vi "Calculate Stuff.vi"(0 "RTD in":dbl[](array[numeric]), 1 "Compressor Displacement Volume":dbl, 3 "Power (Need Input Module)":dbl format="%#_13g", 5 "TC in":dbl[](array[numeric]), 7 "Units":string(combo), 9 "P in":dbl[](array[numeric]), 11 "mdot in":dbl[](array[numeric]), 12 "Compressor Rotational Speed (need input module)":dbl, 14 "fluid name":u16(ring)=17 items=["AIR.MIX", "AMARILLO.MIX", "EKOFISK.MIX", "GLFCOAST.MIX", "HIGHCO2.MIX", "HIGHN2.MIX", "NGSAMPLE.MIX", "R401A.MIX", "R401B.MIX", "R401C.MIX", "R402A.MIX", "R402B.MIX", "R403A.MIX", "R403B.MIX", "R405A.MIX", "R406A.MIX", "R407A.MIX", "R407B.MIX", "R407C.MIX", "R407D.MIX", "R407E.MIX", "R408A.MIX", "R409A.MIX", "R409B.MIX", "R410A.PPF", "R410B.MIX", "R411A.MIX", "R411B.MIX", "R412A.MIX", "R413A.MIX", "R414B.MIX", "R415A.MIX", "R415B.MIX", "R416A.MIX", "R417A.MIX", "R417B.MIX", "R417C.MIX", "R418A.MIX", "R419A.MIX", "R419B.MIX", "R420A.MIX", "R421A.MIX", "R421B.MIX", "R422A.MIX", "R422B.MIX", "R422C.MIX", "R422D.MIX", "R422E.MIX", "R423A.MIX", "R424A.MIX", "R425A.MIX", "R426A.MIX", "R427A.MIX", "R428A.MIX", "R429A.MIX", "R430A.MIX", "R431A.MIX", "R432A.MIX", "R433A.MIX", "R433B.MIX", "R433C.MIX", "R434A.MIX", "R435A.MIX", "R436A.MIX", "R436B.MIX", "R437A.MIX", "R438A.MIX", "R439A.MIX", "R440A.MIX", "R441A.MIX", "R442A.MIX", "R443A.MIX", "R444A.MIX", "R444B.MIX", "R445A.MIX", "R446A.MIX", "R447A.MIX", "R448A.MIX", "R449A.MIX", "R449B.MIX", "R450A.MIX", "R451A.MIX", "R451B.MIX", "R452A.MIX", "R452B.MIX", "R452C.MIX", "R453A.MIX", "R454A.MIX", "R454B.MIX", "R454C.MIX", "R455A.MIX", "R456A.MIX", "R457A.MIX", "R459A.MIX", "R459B.MIX", "R460A.MIX", "R460B.MIX", "R500.MIX", "R501.MIX", "R502.MIX", "R503.MIX", "R504.MIX", "R507A.MIX", "R508A.MIX", "R508B.MIX", "R509A.MIX", "R510A.MIX", "R511A.MIX", "R512A.MIX", "R513A.MIX", "R513B.MIX", "R515A.MIX", "ammonia.fld", "butane.fld", "ethane.fld", "propane.fld", "R11.fld", "R113.fld", "R114.fld", "R115.fld", "R116.fld", "R12.fld", "R123.fld", "R124.fld", "R125.fld", "R13.fld", "R134a.fld", "R14.fld", "R141b.fld", "R142b.fld", "R143a.fld", "R152a.fld", "R161.fld", "R21.fld", "R218.fld", "R22.fld", "R227ea.fld", "R23.fld", "R236ea.fld", "R236fa.fld", "R245ca.fld", "R245fa.fld", "R32.fld", "R41.fld", "R1216.fld", "RC318.fld", "water.fld", "1butene.fld", "acetone.fld", "argon.fld", "benzene.fld", "c1cc6.fld", "c2butene.fld", "c3cc6.fld", "c4f10.fld", "c5f12.fld", "c11.fld", "c12.fld", "cf3i.fld", "CO.fld", "CO2.fld", "COS.fld", "cyclohex.fld", "cyclopen.fld", "cyclopro.fld", "D2.fld", "D2O.fld", "D4.fld", "D5.fld", "D6.fld", "decane.fld", "dee.fld", "dmc.fld", "dme.fld", "ebenzene.fld", "ethanol.fld", "ethylene.fld", "flourine.fld", "H2S.fld", "HCl.fld", "helium.fld", "heptane.fld", "hexane.fld", "hydrogen.fld", "ibutene.fld", "ihexane.fld", "ioctane.fld", "ipentane.fld", "isobutan.fld", "krypton.fld", "MD2M.fld", "MD3M.fld", "MD4M.fld", "MDM.fld", "methane.fld", "methanol.fld", "mlinolea.fld", "mlinolen.fld", "MM.fld", "moleate.fld", "mpalmita.fld", "mstearat.fld", "mxylene.fld", "N2O.fld", "neon.fld", "neopentn.fld", "NF3.fld", "nitrogen.fld", "nonane.fld", "novec649.fld", "octane.fld", "orthohyd.fld", "oxygen.fld", "parahyd.fld", "pentane.fld", "propylen.fld", "propyne.fld", "pxylene.fld", "R365MFC.fld", "R1233zd.fld", "R1234yf.fld", "R1234ze.fld", "RE143a.fld", "RE245cb2.fld", "RE245fa2.fld", "RE347mcc.fld", "sf6.fld", "SO2.fld", "T2butene.fld", "xenon.fld"]) -> (4 "Calculated Values":dbl[](array[numeric]))   [LabVIEW 2017]
panel:
  out "Capacity":dbl
  out "DT subcool":dbl
  out "DT superheat":dbl
  out "Isentropic Efficiency":dbl
  out "Volumetric Efficiency":dbl
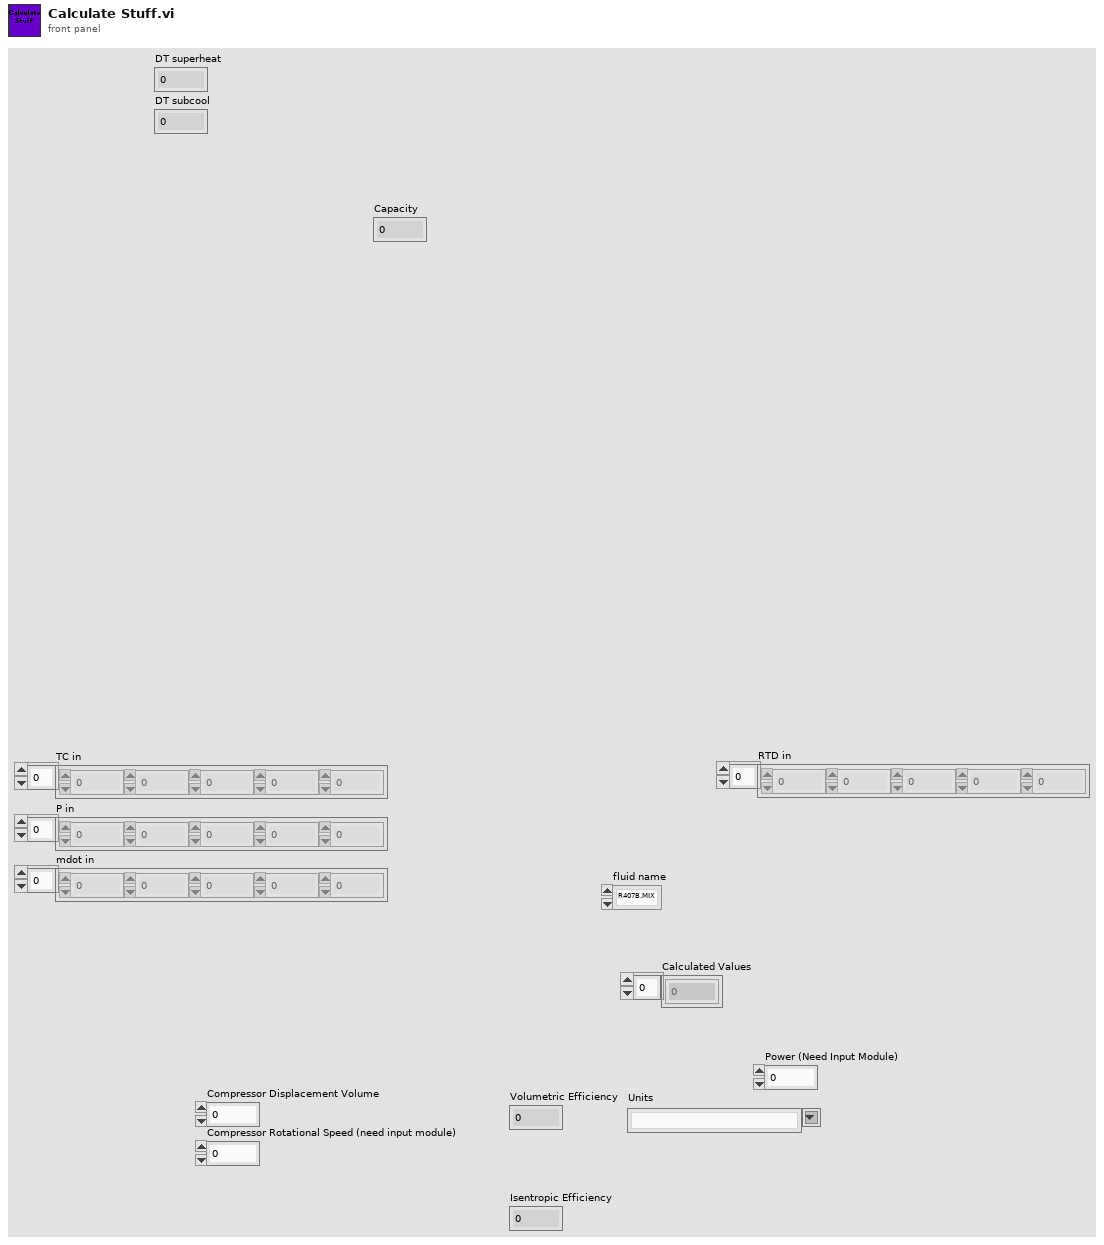
[diagram p1: front panel]
types:
  T1 = enum16{"0", "PS", "HS", "T", "P", "TP", "TH", "TS", "PH", "PQ", "TQ"}
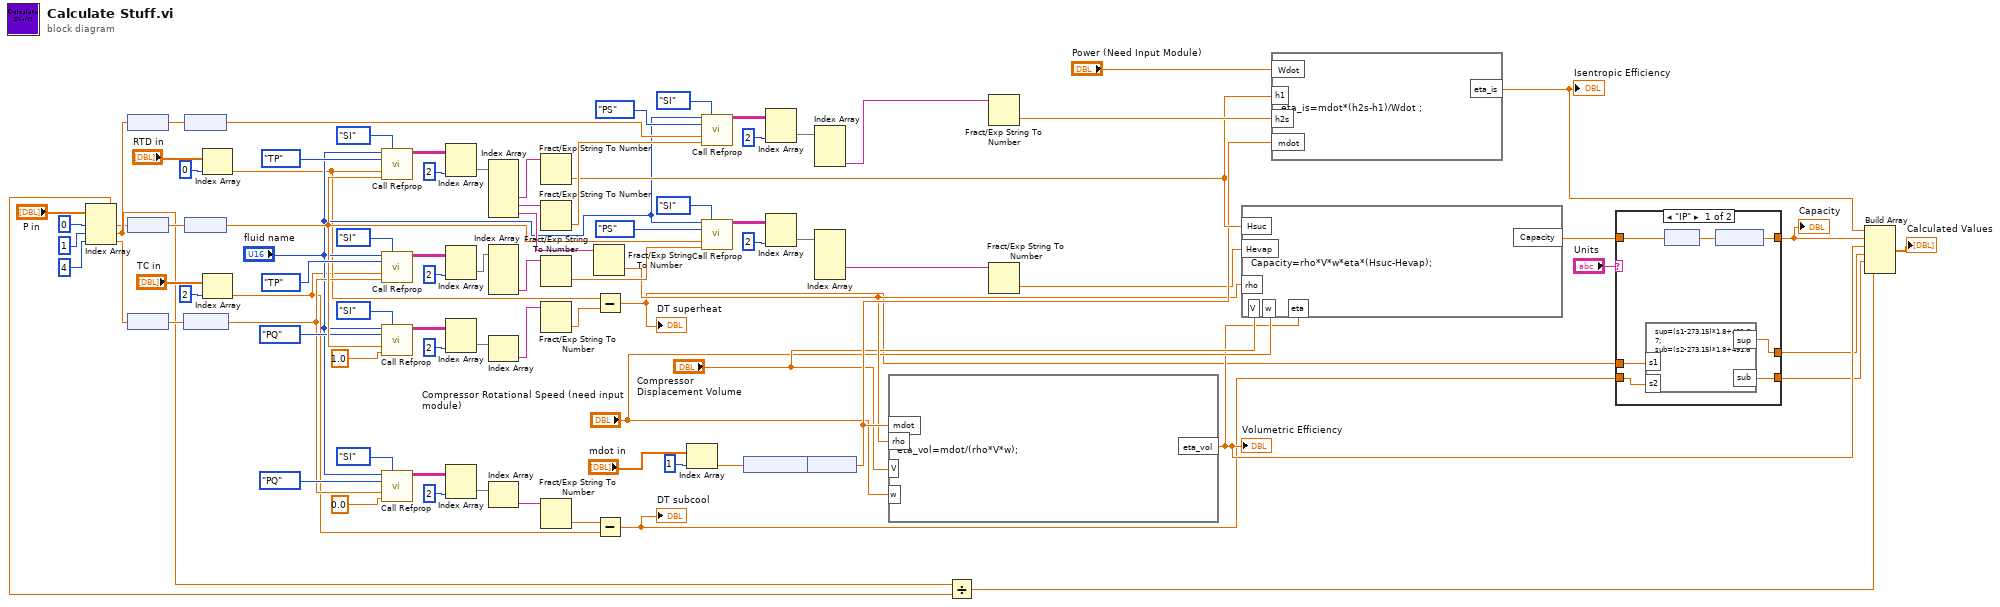
[diagram p0: block diagram]
diagram:
  n1 = Index Array(array="P in", index #1=0 ("index"), index #2=1 ("index"), index #3=4 ("index")) -> (element #1=w2:dbl, element #2=w3:dbl, element #3=w24:dbl)
  n2 = node(w3) -> (w86:dbl[unit])
  n3 = node(w2) -> (w85:dbl[unit])
  n4 = node(w24) -> (w25:dbl[unit])
  n5 = node(w25) -> (w23:dbl)
  n6 = node(w86) -> (w87:dbl)
  n7 = node(w85) -> (w48:dbl)
  n8 = Index Array(array="RTD in", index=0) -> (element=w12:dbl)
  n9 = Index Array(array="TC in", index=2) -> (element=w11:dbl)
  n10 = call "Call Refprop.vi"("fluid name"="fluid name", "units"=enum16{"SI", "IP"}."SI", "InpCode"=T1."TP", "output_1"=w12, "output_2"=w48) -> ("data"=w75:string[][])  [unwired: 6 in, 4 out]
  n11 = call "Call Refprop.vi"("fluid name"="fluid name", "units"=enum16{"SI", "IP"}."SI", "InpCode"=T1."TP", "output_1"=w11, "output_2"=w23) -> ("data"=w63:string[][])  [unwired: 6 in, 4 out]
  n12 = call "Call Refprop.vi"("fluid name"="fluid name", "units"=enum16{"SI", "IP"}."SI", "InpCode"=T1."PQ", "output_1"=w48, "output_2"=1.0) -> ("data"=w45:string[][])  [unwired: 6 in, 4 out]
  n13 = call "Call Refprop.vi"("fluid name"="fluid name", "units"=enum16{"SI", "IP"}."SI", "InpCode"=T1."PQ", "output_1"=w23, "output_2"=0.0) -> ("data"=w38:string[][])  [unwired: 6 in, 4 out]
  n14 = Index Array(array=w75, index (col)=2 ("disabled index (col)")) -> (element=w76:string[])  [unwired: 1 in]
  n15 = Index Array(array=w63, index (col)=2 ("disabled index (col)")) -> (element=w61:string[])  [unwired: 1 in]
  n16 = Index Array(array=w45, index (col)=2 ("disabled index (col)")) -> (element=w43:string[])  [unwired: 1 in]
  n17 = Index Array(array=w38, index (col)=2 ("disabled index (col)")) -> (element=w36:string[])  [unwired: 1 in]
  n18 = Index Array(array=w76) -> (element #3=w84:string, element #4=w77:string, element #5=w83:string)  [unwired: 5 in, 2 out]
  n19 = Index Array(array=w61) -> (element #4=w59:string)  [unwired: 4 in, 3 out]
  n20 = Index Array(array=w43) -> (element=w42:string)  [unwired: 1 in]
  n21 = Index Array(array=w36) -> (element=w35:string)  [unwired: 1 in]
  n22 = Fract/Exp String To Number(string=w84) -> (number=w67:dbl)  [unwired: 3 in, 1 out]
  n23 = Fract/Exp String To Number(string=w77) -> (number=w78:dbl)  [unwired: 3 in, 1 out]
  n24 = Fract/Exp String To Number(string=w59) -> (number=w58:dbl)  [unwired: 3 in, 1 out]
  n25 = Fract/Exp String To Number(string=w42) -> (number=w41:dbl)  [unwired: 3 in, 1 out]
  n26 = Fract/Exp String To Number(string=w35) -> (number=w34:dbl)  [unwired: 3 in, 1 out]
  n27 = Fract/Exp String To Number(string=w83) -> (number=w51:dbl)  [unwired: 3 in, 1 out]
  n28 = Subtract(x=w12, y=w41) -> (x-y=w7:dbl)
  "DT superheat" <- w7
  n29 = Subtract(x=w34, y=w11) -> (x-y=w5:dbl)
  "DT subcool" <- w5
  n30 = Index Array(array="mdot in", index=1) -> (element=w20:dbl)
  n31 = call "Call Refprop.vi"("fluid name"="fluid name", "units"=enum16{"SI", "IP"}."SI", "InpCode"=T1."PS", "output_1"=w87, "output_2"=w78) -> ("data"=w79:string[][])  [unwired: 6 in, 4 out]
  n32 = call "Call Refprop.vi"("fluid name"="fluid name", "units"=enum16{"SI", "IP"}."SI", "InpCode"=T1."PS", "output_1"=w48, "output_2"=w58) -> ("data"=w56:string[][])  [unwired: 6 in, 4 out]
  n33 = node(w20) -> (w70:dbl[unit])
  n34 = Index Array(array=w79, index (col)=2 ("disabled index (col)")) -> (element=w80:string[])  [unwired: 1 in]
  n35 = Index Array(array=w56, index (col)=2 ("disabled index (col)")) -> (element=w54:string[])  [unwired: 1 in]
  n36 = node(w70) -> (w66:dbl)
  n37 = Index Array(array=w80) -> (element #3=w81:string)  [unwired: 3 in, 2 out]
  n38 = Index Array(array=w54) -> (element #3=w53:string)  [unwired: 4 in, 3 out]
  n39 = formula code="eta_vol=mdot/(rho*V*w);"("mdot"=w66, "rho"=w51, "V"="Compressor Displacement Volume", "w"="Compressor Rotational Speed (need input module)") -> ("eta_vol"=w13:dbl)
  "Volumetric Efficiency" <- w13
  n40 = Divide(x=w3, y=w2) -> (x/y=w1:dbl)
  n41 = Fract/Exp String To Number(string=w81) -> (number=w82:dbl)  [unwired: 3 in, 1 out]
  n42 = Fract/Exp String To Number(string=w53) -> (number=w52:dbl)  [unwired: 3 in, 1 out]
  n43 = formula code="Capacity=rho*V*w*eta*(Hsuc-Hevap);"("rho"=w51, "V"="Compressor Displacement Volume", "w"="Compressor Rotational Speed (need input module)", "Hsuc"=w67, "Hevap"=w52, "eta"=w13) -> ("Capacity"=w9:dbl)
  n44 = formula code="eta_is=mdot*(h2s-h1)/Wdot ;"("h2s"=w82, "h1"=w67, "mdot"=w66, "Wdot"="Power (Need Input Module)") -> ("eta_is"=w18:dbl)
  "Isentropic Efficiency" <- w18
  n45 = case shown="\"IP\"" "Units" {
    tunnel: w9 -> [w94 w97]
    tunnel: [w92 w97] -> w8
    tunnel: w7 -> [w90 w96]
    tunnel: [w88 w96] -> w6
    tunnel: w5 -> [w91 w95]
    tunnel: [w89 w95] -> w4
    frame "IP" {
      n46 = formula code="sup=(s1-273.15)*1.8+491.67;\nsub=(s2-273.15)*1.8+491.67;"("s1"=w90, "s2"=w91) -> ("sup"=w88:dbl, "sub"=w89:dbl)
      n47 = node(w94) -> (w93:dbl[unit])
      n48 = node(w93) -> (w92:dbl)
    }
    frame "SI", Default {
    }
  }
  "Capacity" <- w8
  n49 = Build Array(w18, w8, w13, w6, w4, w1) -> (→"Calculated Values":dbl[])
